vi "Modbus.StopServers.vi"(8 "error in (no error)":errorcluster) -> (0 "error out":errorcluster)   [LabVIEW 2019, in "Modbus.lvlib"]
uses:
  Modbus.lvlib
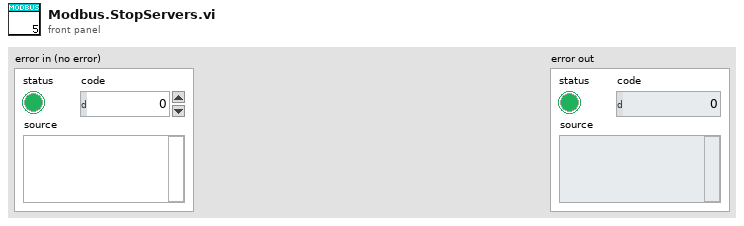
[diagram p1: front panel]
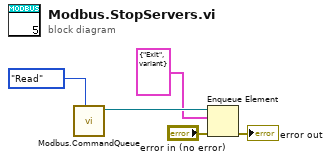
[diagram p0: block diagram]
diagram:
  n1 = call "Modbus.CommandQueue.vi"("OP"=enum16{"Read", "Write"}."Read") -> ("queue OUT"=w4:refnum<queue>)  [unwired: 10 in]
  n2 = Enqueue Element(queue=w4, element=cluster{"Command":string, "Data":variant} {"Command"="Exit", "Data"=variant}, error in (no error)="error in (no error)") -> (error out=→"error out":errorcluster)  [unwired: 1 in, 2 out]
